vi "Светофор у общаги.vi"() -> ()   [LabVIEW 2021]
uses:
  Control 1-.ctl
panel:
  in  "stop":bool
  out "Время":i32
  in  "Вызов":bool
  out "Пешеходы":T1
  out "Машины":T2
  out "Состояние":T3
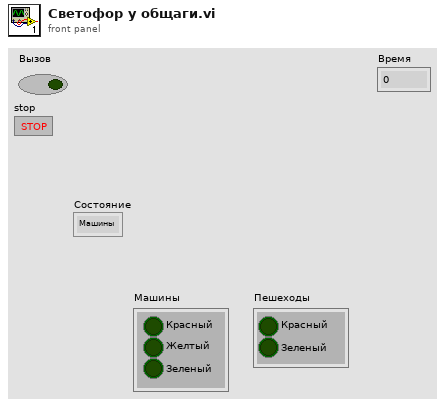
[diagram p1: front panel]
types:
  T1 = typedef "Пешеходы.ctl" = cluster{"Красный":bool, "Зеленый":bool}
  T2 = typedef "Машины.ctl" = cluster{"Красный":bool, "Желтый":bool, "Зеленый":bool}
  T3 = typedef "Control 1-.ctl" = enum16{"Машины", "Желтый1", "Пешеходы", "Желтый2"}
  T4 = cluster{"Красный":bool, "Желтый":bool, "Зеленый":bool}
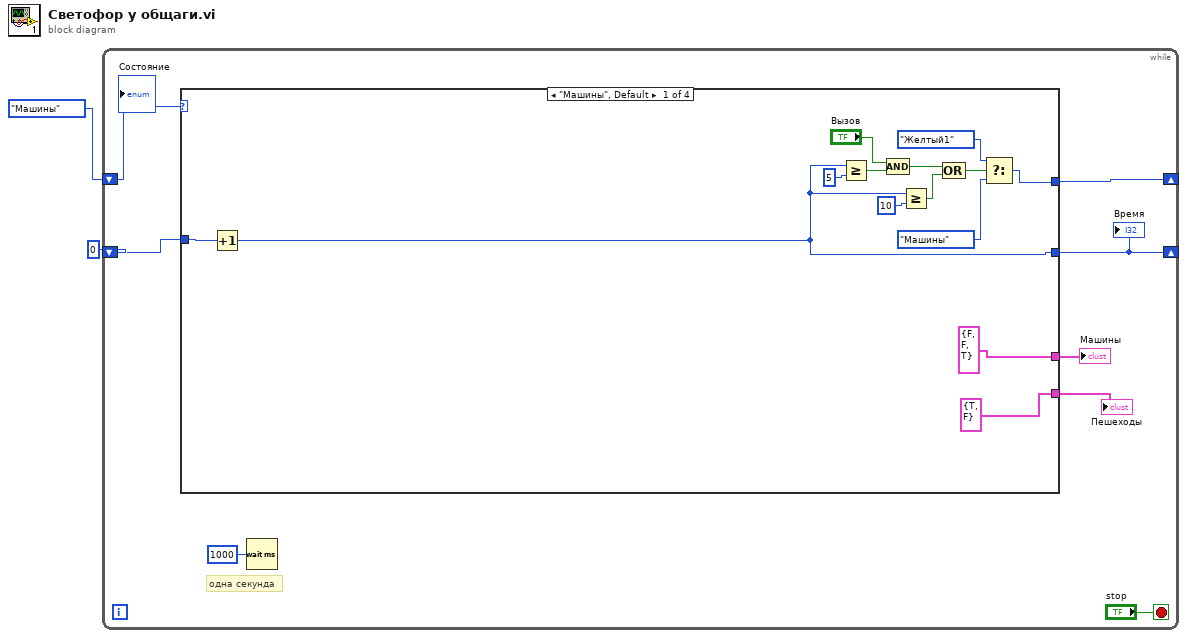
[diagram p0: block diagram]
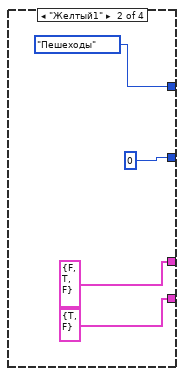
[diagram p2: hidden frame]
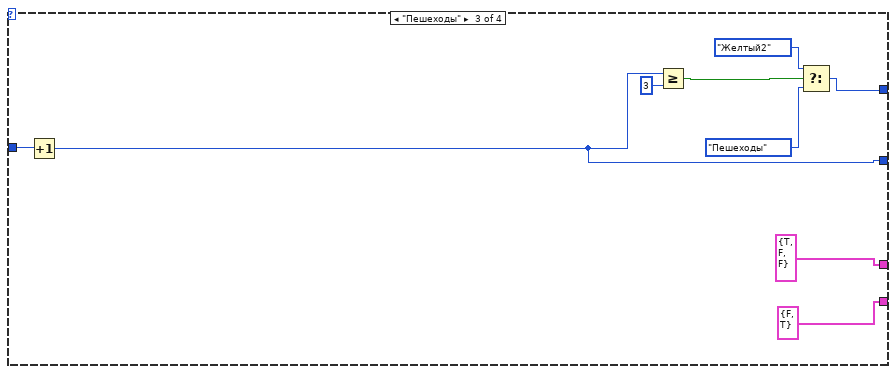
[diagram p3: hidden frame]
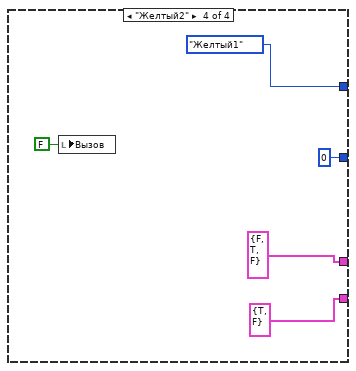
[diagram p4: hidden frame]
diagram:
  n1 = while {
    shift-right: [w7] -> _
    shift-left: Control_1-."Машины" ("Состояние") -> [w10]
    shift-right: [w6] -> _
    shift-left: 0 -> [w8]
    stop <- "stop" stop-if-true
    # "одна секунда"
    n2 = case shown="\"Машины\", Default" w10 {
      tunnel: w8 -> [w14 _ w34 _]
      tunnel: [w15 Control_1-."Пешеходы" ("Состояние") w33 Control_1-."Желтый1" ("Состояние")] -> w7
      tunnel: [w11 0 w29 0] -> w6
      tunnel: [T4 {"Красный"=FALSE, "Желтый"=FALSE, "Зеленый"=TRUE} ("Машины") T4 {"Красный"=FALSE, "Желтый"=TRUE, "Зеленый"=FALSE} ("Машины") T4 {"Красный"=TRUE, "Желтый"=FALSE, "Зеленый"=FALSE} ("Машины") T4 {"Красный"=FALSE, "Желтый"=TRUE, "Зеленый"=FALSE} ("Машины")] -> w5
      tunnel: [cluster{"Красный":bool, "Зеленый":bool} {"Красный"=TRUE, "Зеленый"=FALSE} ("Пешеходы") cluster{"Красный":bool, "Зеленый":bool} {"Красный"=TRUE, "Зеленый"=FALSE} ("Пешеходы") cluster{"Красный":bool, "Зеленый":bool} {"Красный"=FALSE, "Зеленый"=TRUE} ("Пешеходы") cluster{"Красный":bool, "Зеленый":bool} {"Красный"=TRUE, "Зеленый"=FALSE} ("Пешеходы")] -> w4
      frame "Машины", Default {
        n3 = Increment(x=w14) -> (x+1=w11:i32)
        n4 = Greater Or Equal?(x=w11, y=5) -> (x >= y?=w21:bool)
        n5 = Compound Arithmetic op=AND("Вызов", w21) -> (w20:bool)
        n6 = Greater Or Equal?(x=w11, y=10) -> (x >= y?=w19:bool)
        n7 = Compound Arithmetic op=OR(w20, w19) -> (w18:bool)
        n8 = Select(t=Control_1-."Желтый1" ("Состояние"), s=w18, f=Control_1-."Машины" ("Состояние")) -> (s? t:f=w15:T3)
      }
      frame "Желтый1" {
      }
      frame "Пешеходы" {
        n9 = Increment(x=w34) -> (x+1=w29:i32)
        n10 = Greater Or Equal?(x=w29, y=3) -> (x >= y?=w30:bool)
        n11 = Select(t=Control_1-."Желтый2" ("Состояние"), s=w30, f=Control_1-."Пешеходы" ("Состояние")) -> (s? t:f=w33:T3)
      }
      frame "Желтый2" {
        n12 = local write "Вызов"(FALSE ("Вызов")) -> ()
      }
    }
    "Машины" <- w5
    "Пешеходы" <- w4
    "Время" <- w6
    n13 = Wait (ms)(milliseconds to wait=u32 1000) -> ()  [unwired: 1 out]
    "Состояние" <- w10
  }
